vi "Pay to String.vi"(8 "error in":errorcluster, 11 "payload":u8[](array[numeric])=[3, 0, 7, 0, 255] format="%x") -> (0 "error out":errorcluster, 2 "Extra Value":u8, 3 "State":u8 format="%x")   [LabVIEW 2023, in "Decoder.lvlib"]
doc: "Decode the frame recieved and determine if it is a valid option so send the comand to the FPGA"
uses:
  Decoder.lvlib
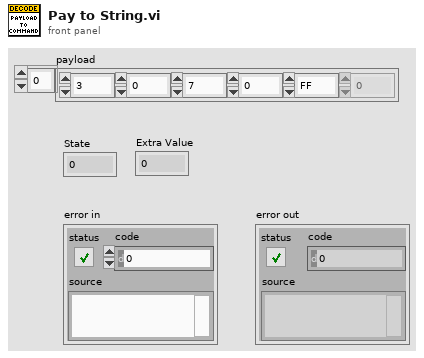
[diagram p1: front panel]
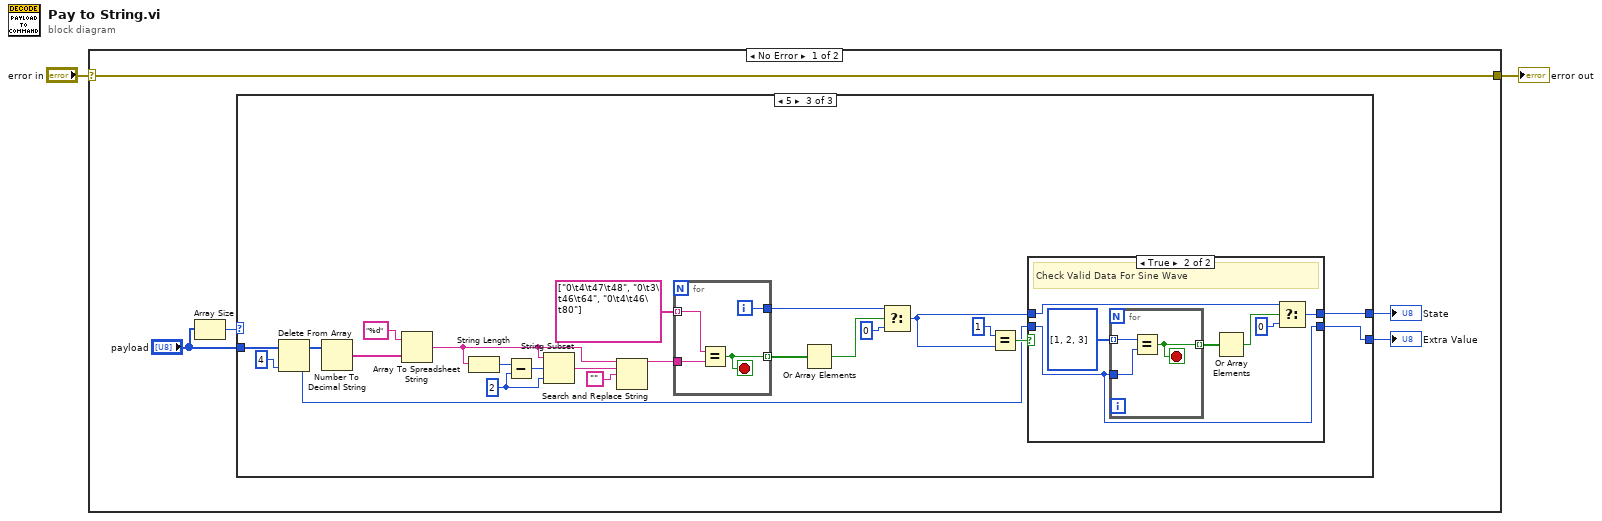
[diagram p0: block diagram]
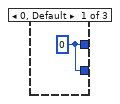
[diagram p2: hidden frame]
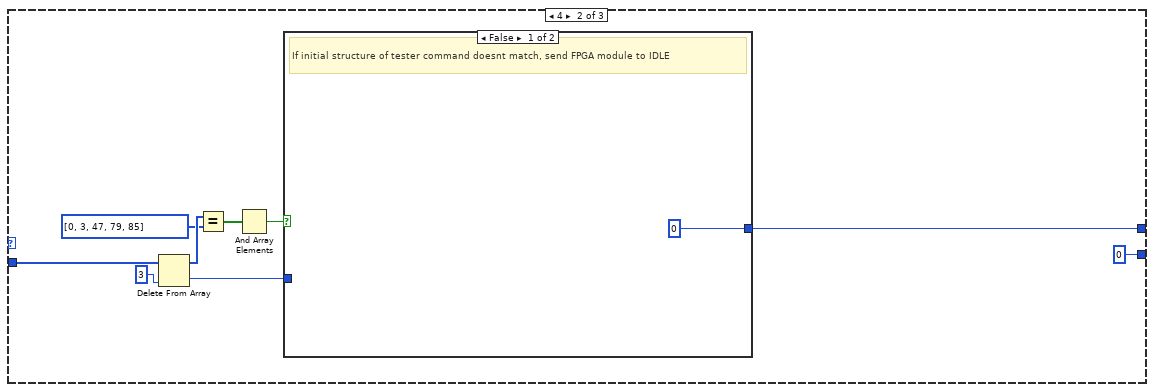
[diagram p3: hidden frame]
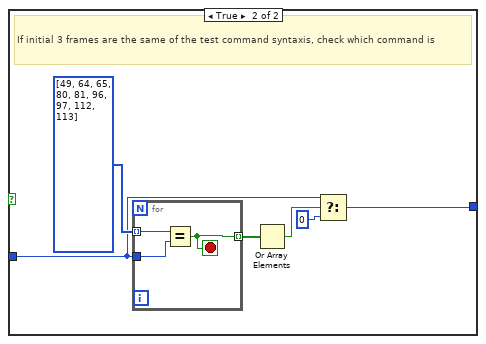
[diagram p4: hidden frame]
diagram:
  n1 = case shown="No Error" "error in" {
    selector: "error in" -> [w7 w67]
    tunnel: [w7 w67] -> w1
    frame No Error {
      n2 = Array Size(array="payload") -> (size(s)=w5:i32)
      n3 = case shown="5" w5 {
        tunnel: "payload" -> [_ w17 w40]
        tunnel: [w8 w9 w28] -> w4
        tunnel: [w8 u8 0 ("Numeric 3") w29] -> w3
        frame 0, Default {
          w8 = u8 0 ("Numeric 2")
        }
        frame 4 {
          n4 = Delete From Array(array=w17, index=3 ("index 2")) -> (deleted portion=w11:u8, array with subset deleted=w15:u8[])  [unwired: 1 in]
          n5 = Equal?(x=w15, y=u8[] [0, 3, 47, 79, 85] ("payload 3")) -> (x = y?=w13:bool[])
          n6 = And Array Elements(Boolean array=w13) -> (logical AND=w10:bool)
          n7 = case shown="False" w10 {
            tunnel: w11 -> [_ w21]
            tunnel: [u8 0 ("f") w20] -> w9
            frame False {
              # "If initial structure of tester command doesnt match, send FPGA module to IDLE"
            }
            frame True {
              # "If initial 3 frames are the same of the test command syntaxis, check which command is"
              n8 = for {
                tunnel: u8[] [49, 64, 65, 80, 81, 96, 97, 112, 113] -> [w27] mode=indexing
                tunnel: w21 -> [w25]
                tunnel: [w26] -> w23 mode=indexing
                stop <- w26 stop-if-true
                n9 = Equal?(x=w27, y=w25) -> (x = y?=w26:bool)
              }
              n10 = Or Array Elements(Boolean array=w23) -> (logical OR=w22:bool)
              n11 = Select(t=w21, s=w22, f=u8 0) -> (s? t:f=w20:u8)
            }
          }
        }
        frame 5 {
          w48 = 2 ("y")
          n12 = Delete From Array(array=w40, index=4 ("index 2")) -> (deleted portion=w30:u8, array with subset deleted=w39:u8[])  [unwired: 1 in]
          n13 = Number To Decimal String(number=w39) -> (decimal integer string=w37:string[])  [unwired: 1 in]
          n14 = Array To Spreadsheet String(array=w37, 3:"%d" ("format string")) -> (spreadsheet string=w46:string)  [unwired: 1 in]
          n15 = String Length(string=w46) -> (length=w49:i32)
          n16 = Subtract(x=w49, y=w48) -> (x-y=w47:i32)
          n17 = String Subset(string=w46, offset (0)=w47, length (rest)=w48) -> (substring=w44:string)
          n18 = Search and Replace String(input string=w46, search string=w44, replace string="") -> (result string=w42:string)  [unwired: 5 in, 3 out]
          n19 = for {
            tunnel: string[] ["0\t4\t47\t48", "0\t3\t46\t64", "0\t4\t46\t80"] -> [w66] mode=indexing
            tunnel: w42 -> [w65]
            tunnel: [w64] -> w38 mode=indexing
            tunnel: [w63] -> w35
            i -> [w63]
            stop <- w64 stop-if-true
            n20 = Equal?(x=w66, y=w65) -> (x = y?=w64:bool)
          }
          n21 = Or Array Elements(Boolean array=w38) -> (logical OR=w36:bool)
          n22 = Select(t=w35, s=w36, f=0) -> (s? t:f=w31:i32)
          n23 = Equal?(x=1, y=w31) -> (x = y?=w32:bool)
          n24 = case shown="True" w32 {
            tunnel: w31 -> [w52 w56]
            tunnel: [w52 w54] -> w28
            tunnel: w30 -> [w51 w53]
            tunnel: [w51 w53] -> w29
            frame False {
            }
            frame True {
              # "Check Valid Data For Sine Wave"
              n25 = for {
                tunnel: w53 -> [w62]
                tunnel: u8[] [1, 2, 3] -> [w61] mode=indexing
                tunnel: [w60] -> w58 mode=indexing
                stop <- w60 stop-if-true
                n26 = Equal?(x=w61, y=w62) -> (x = y?=w60:bool)
              }
              n27 = Or Array Elements(Boolean array=w58) -> (logical OR=w57:bool)
              n28 = Select(t=w56, s=w57, f=u8 0) -> (s? t:f=w54:i32)
            }
          }
        }
      }
      "State" <- w4
      "Extra Value" <- w3
    }
    frame Error {
    }
  }
  "error out" <- w1
